vi "OP300ZP_Param_ConfZENplusOP100.vi"(8 "errin":errorcluster, 10 "Chaîne":string, 11 "pathin":path) -> (0 "errout":errorcluster, 3 "VISA OUT":T1)   [LabVIEW 2020]
uses:
  <vilib>/Utility/config.llb/Read Key (String).vi
  <vilib>/Utility/config.llb/NI_LVConfig.lvlib
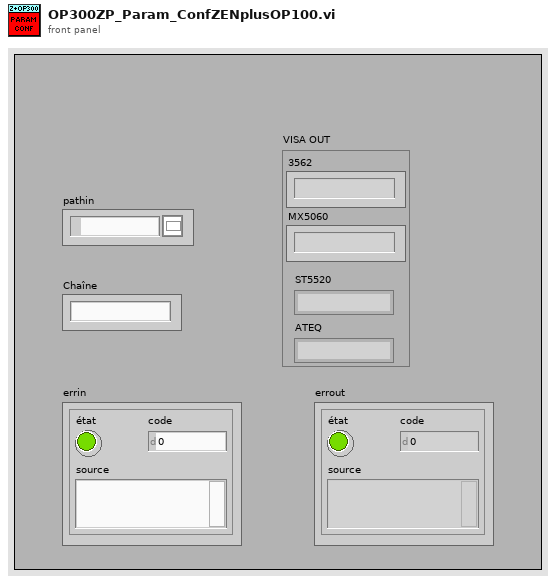
[diagram p1: front panel]
types:
  T1 = cluster{"3562":string, "MX5060":string, "ST5520":string, "ATEQ":string}
  T2 = typedef "NI_LVConfig.lvlib/Config Data RefNum.ctl" = refnum<k1>
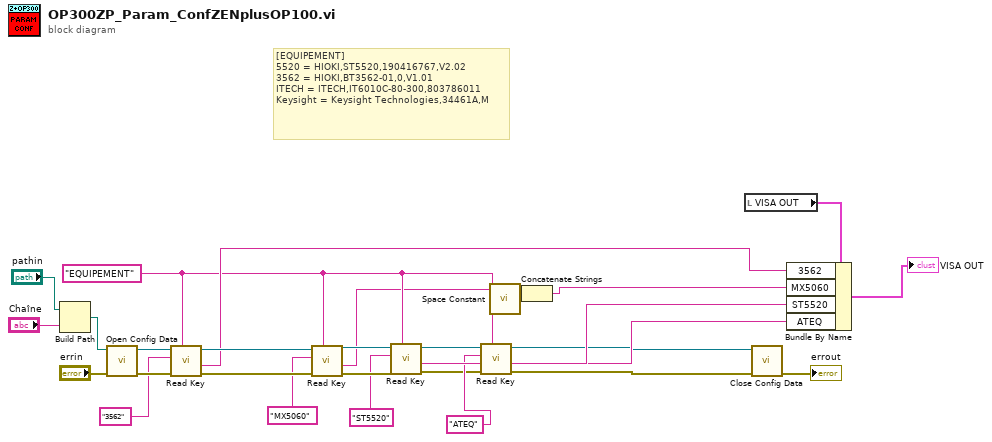
[diagram p0: block diagram]
diagram:
  w7 = "EQUIPEMENT" ("section")
  # "[EQUIPEMENT]\n5520 = HIOKI,ST5520,190416767,V2.02\n3562 = HIOKI,BT3562-01,0,V1.01\nITECH = ITECH,IT6010C-80-300,803786011\nKeysight = Keysight Technologies,34461A,M"
  n1 = Build Path(base path="pathin", name or relative path="Chaîne") -> (appended path=w25:path)
  n2 = call <vilib>:"Open Config Data.vi"("error in (no error)"="errin", "configuration file path"=w25) -> ("error out"=w27:errorcluster, "refnum"=w28:T2)  [unwired: 7 in, 1 out]
  n3 = call-poly <vilib>:"Read Key.vi"("section"=w7, "error in (no error)"=w27, "key"="3562", "refnum"=w28) -> ("error out"=w22:errorcluster, "value"=w17:string, "refnum out"=w24:T2)  [unwired: 4 in, 1 out]
  n4 = call-poly <vilib>:"Read Key.vi"("section"=w7, "error in (no error)"=w22, "key"="MX5060", "refnum"=w24) -> ("error out"=w13:errorcluster, "value"=w3:string, "refnum out"=w12:T2)  [unwired: 4 in, 1 out]
  n5 = call-poly <vilib>:"Read Key.vi"("section"=w7, "error in (no error)"=w13, "key"="ST5520", "refnum"=w12) -> ("error out"=w9:errorcluster, "value"=w16:string, "refnum out"=w5:T2)  [unwired: 4 in, 1 out]
  n6 = call-poly <vilib>:"Read Key.vi"("section"=w7, "error in (no error)"=w9, "key"="ATEQ", "refnum"=w5) -> ("error out"=w8:errorcluster, "value"=w6:string, "refnum out"=w4:T2)  [unwired: 4 in, 1 out]
  n7 = call <vilib>:"Space Constant.vi"() -> ("String"=w2:string)
  n8 = Concatenate Strings(w3, w2) -> (w1:string)
  n9 = local read "VISA OUT"() -> (w18:T1)
  n10 = call <vilib>:"Close Config Data.vi"("error in (no error)"=w8, "refnum"=w4) -> ("error out"=→"errout":errorcluster)  [unwired: 8 in, 1 out]
  n11 = Bundle By Name(cluster=w18, "3562"=w17, "MX5060"=w1, "ST5520"=w16, "ATEQ"=w6) -> (→"VISA OUT":T1)
